vi "el_instrumento_virtual_con_otro_nombre.vi"() -> ()   [LabVIEW 2009]
uses:
  <vilib>/Analysis/3filter.llb/Butterworth Filter (DBL).vi
  <vilib>/Analysis/NI_AALBase.lvlib
panel:
  out "Señal sin filtrar":cluster{"Y":dbl[], "Y":dbl[]}[](graph)
  in  "low cutoff freq: fl":dbl=45.0 format="%0.4f"
  in  "Range Constants":u8[](array[ring])=[1, 1] items=["LJ_rgBIP10V", "LJ_rgBIP1V", "LJ_rgBIPP1V", "LJ_rgBIPP01V"]
  out "Filtrada":cluster{"Y":dbl[], "Y":dbl[]}[](graph)
  in  "Number of Samples":dbl=4000.0
  in  "Scan Rate (Hz)":dbl=10000.0 format="%.3f"
  # "Escoger los dos primeros\nelementos de la lista\npara ajustar el margen\ndinámico (de arriba a abajo,\n 10 V, 1 V, 0,1 V y 0,01 V)."
  # "EJEMPLO CON UN FILTRO PASO BAJO"
  # "Señal filtrada"
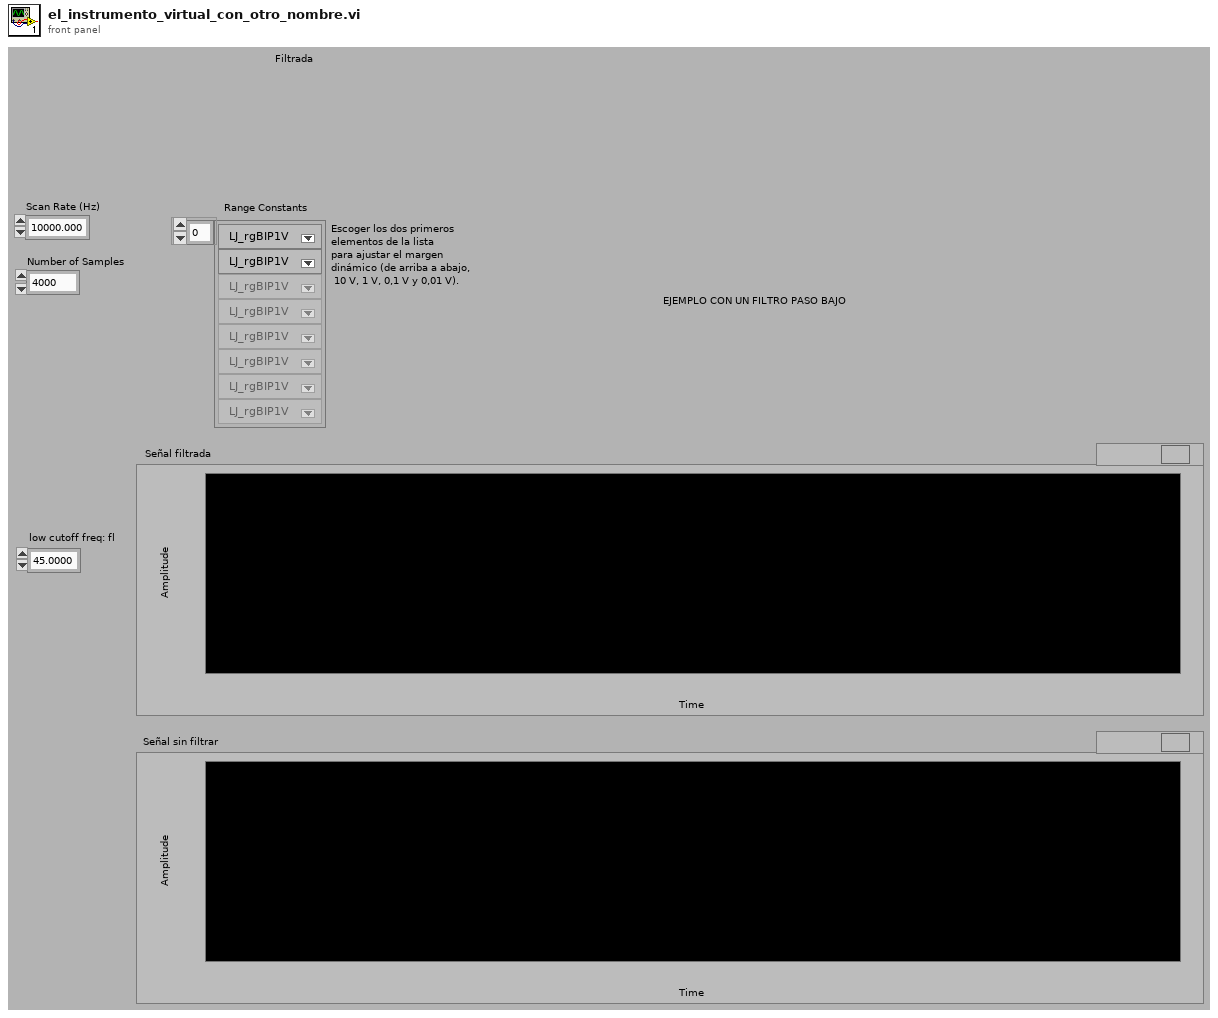
[diagram p1: front panel]
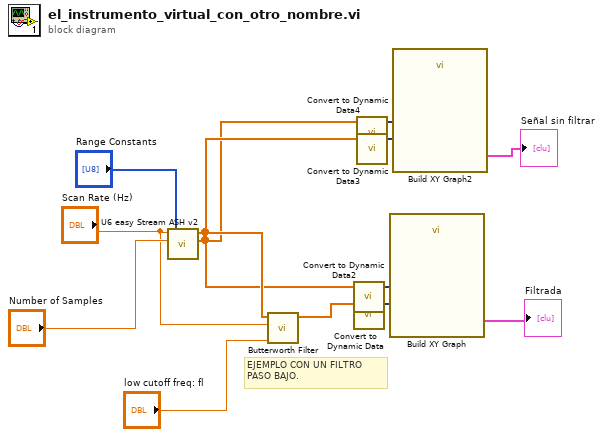
[diagram p0: block diagram]
diagram:
  # "EJEMPLO CON UN FILTRO\nPASO BAJO."
  n1 = call "U6 easy Stream ASH v2.vi"("Range Constants"="Range Constants", "Number of Samples"="Number of Samples", "Scan Rate (Hz)"="Scan Rate (Hz)") -> ("Tiempo"=w2:dbl[], "Señal"=w4:dbl[])  [unwired: 3 in]
  n2 = call-poly <vilib>:"Butterworth Filter.vi"("low cutoff freq: fl"="low cutoff freq: fl", "sampling freq: fs"="Scan Rate (Hz)", "X"=w4) -> ("Filtered X"=w9:dbl[])  [unwired: 5 in, 1 out]
  n3 = call "Convert to Dynamic Data2"("Array"=w2) -> ("Dynamic Data Type"=w11:dynamicdata)  [unwired: 3 in]
  n4 = call "Convert to Dynamic Data"("Array"=w9) -> ("Dynamic Data Type"=w8:dynamicdata)  [unwired: 3 in]
  n5 = call "Convert to Dynamic Data4"("Array"=w2) -> ("Dynamic Data Type"=w1:dynamicdata)  [unwired: 3 in]
  n6 = call "Convert to Dynamic Data3"("Array"=w4) -> ("Dynamic Data Type"=w3:dynamicdata)  [unwired: 3 in]
  n7 = call "Build XY Graph"("Y Input"=w8, "X Input"=w11) -> ("XY Graph"=→"Filtrada":cluster{"Y":dbl[], "Y":dbl[]}[])  [unwired: 8 in, 1 out]
  n8 = call "Build XY Graph2"("Y Input"=w3, "X Input"=w1) -> ("XY Graph"=→"Señal sin filtrar":cluster{"Y":dbl[], "Y":dbl[]}[])  [unwired: 8 in, 1 out]
